vi "HumanExecute.vi"(8 "error in (no error)":errorcluster) -> (0 "error out":errorcluster)   [LabVIEW 2023]
doc: "Execute for Human\n\ninput:\n error in (cluster)\n\noutput:\n error out (cluster)"
uses:
  <vilib>/Rock Robotics/WPI/Joystick/XBox Buttons Indexer.ctl
  <vilib>/Rock Robotics/WPI/Joystick/XBox Axes Indexer.ctl
  <vilib>/Rock Robotics/WPI/ThirdParty/JAS_Junk/TrajLib/VI/BoolCmd_Send_Internal.vi
  <vilib>/Rock Robotics/WPI/ThirdParty/JAS_Junk/TrajLib/VI/BoolCmd_ObtainQueue.vi
  <vilib>/Rock Robotics/Network Tables/NT Write String.vi
  <vilib>/Rock Robotics/WPI/ThirdParty/JAS_Junk/TrajLib/Trajectory_Library.lvlib
  HumanGlobal.vi
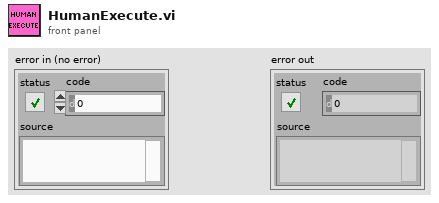
[diagram p1: front panel]
types:
  T1 = typedef "XBox Buttons Indexer.ctl" = enum16{"A", "B", "X", "Y", "Left Bumper", "Right Bumper", "Back", "Start", "Left Joystick", "Right Joystick"}
  T2 = typedef "XBox Axes Indexer.ctl" = enum16{"Left X", "Left Y", "Left Trigger", "Right Trigger", "Right X", "Right Y"}
  T3 = typedef "WPI_JoystickDevRef.ctl" = cluster{"Device":T4}
  T4 = typedef "WPI_JoystickDeviceEnum.ctl" = enum16{"USB 0", "USB 1", "USB 2", "USB 3", "USB 4", "USB 5"}
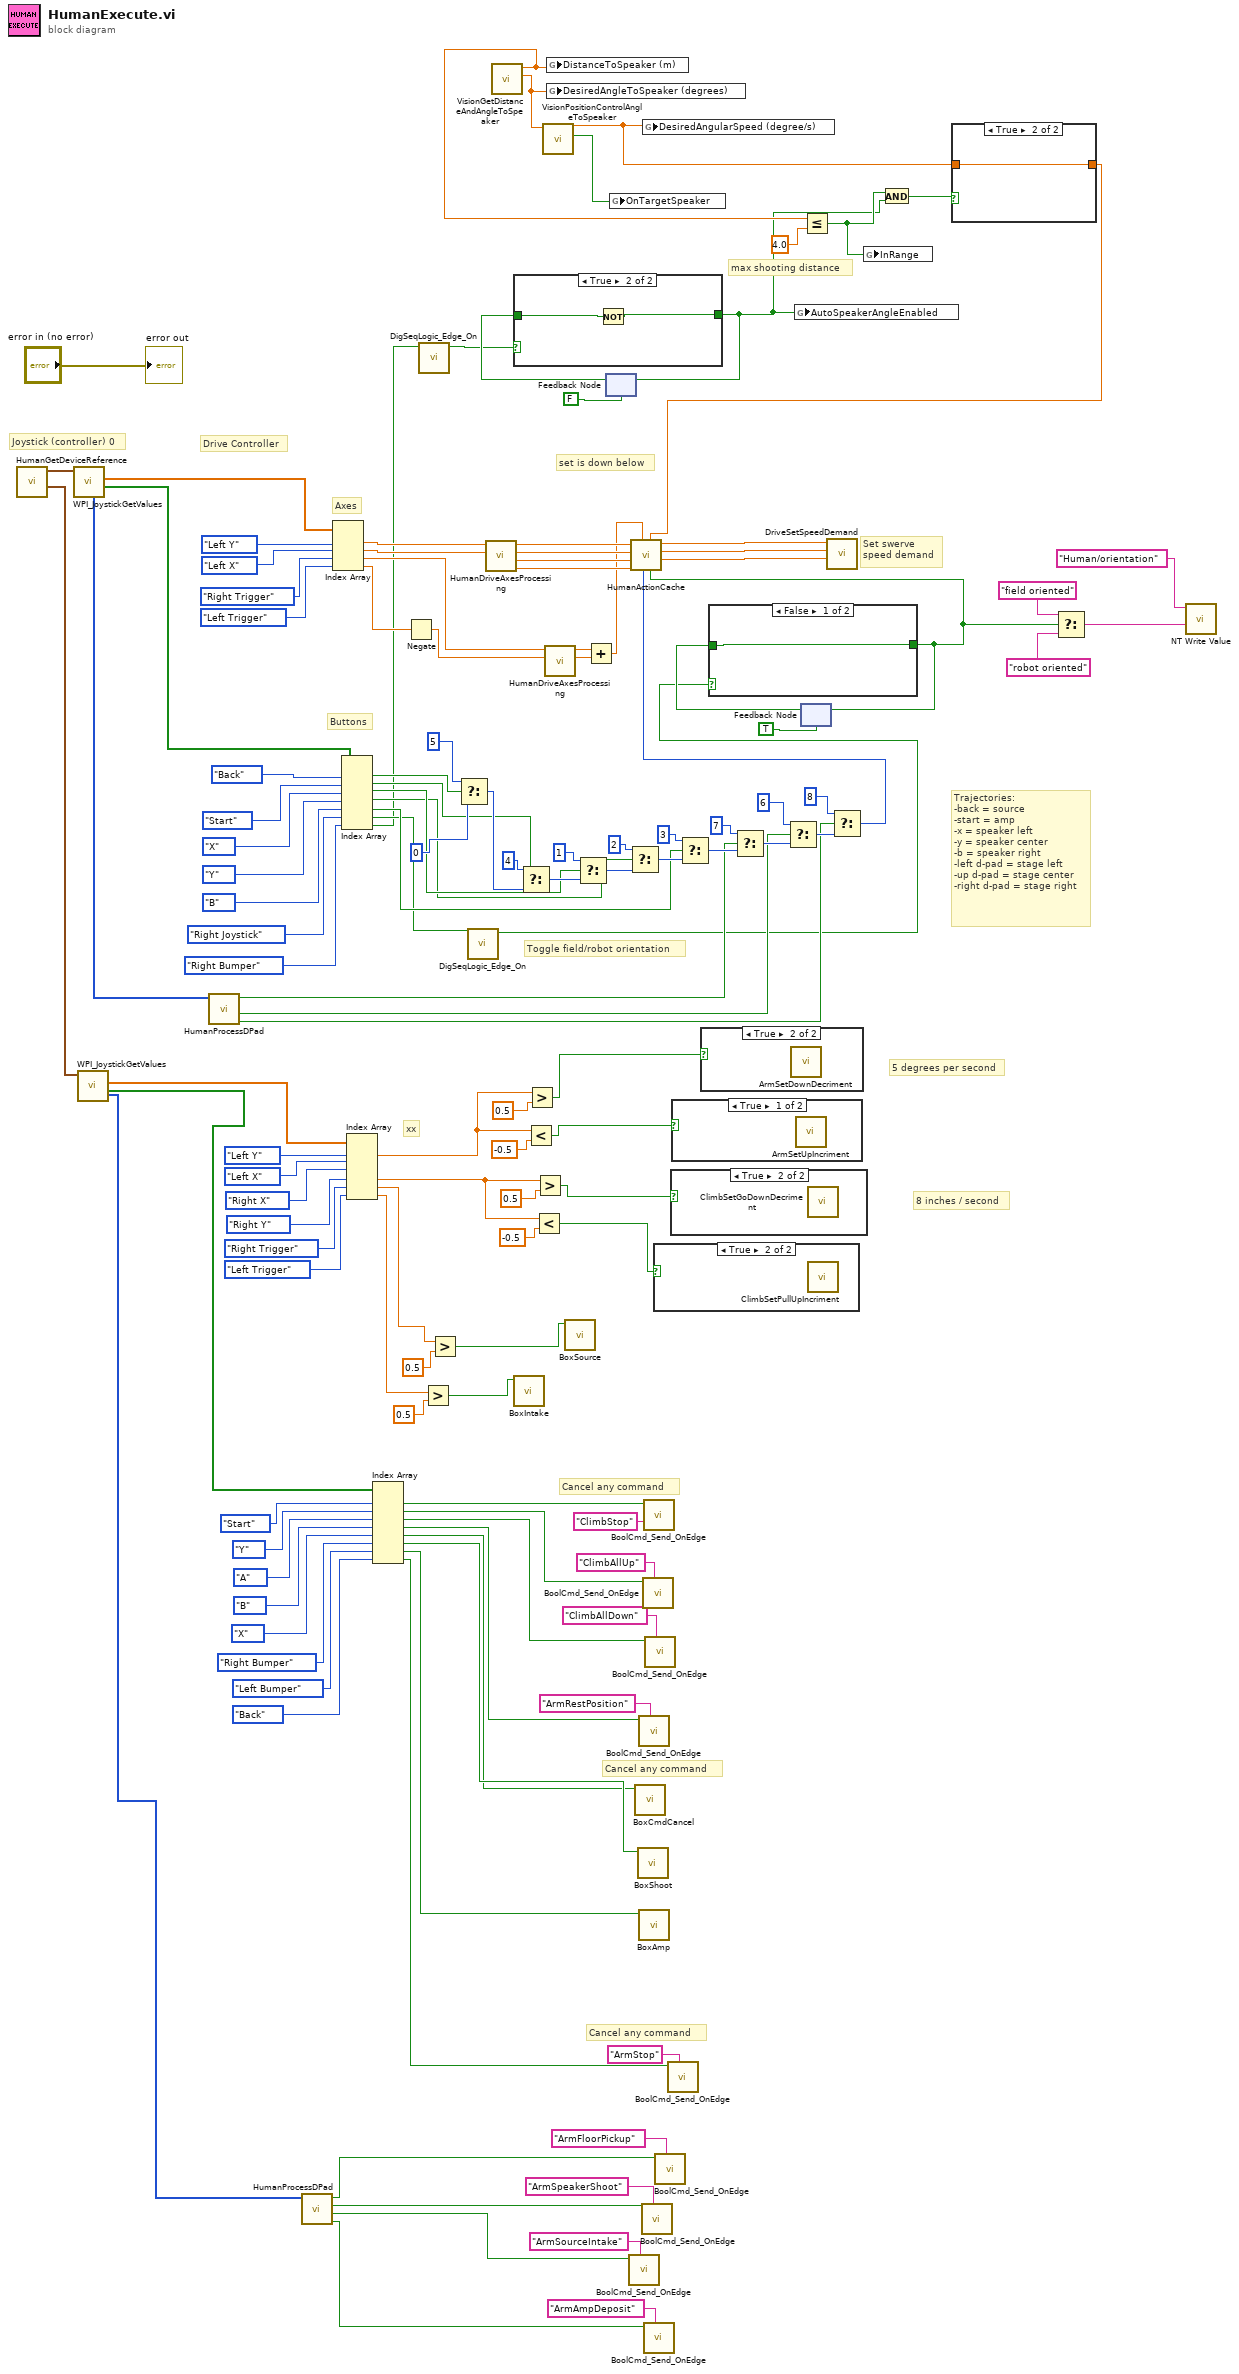
[diagram p0: block diagram]
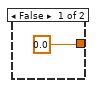
[diagram p3: hidden frame]
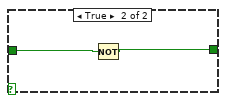
[diagram p4: hidden frame]
diagram:
  # "max shooting distance"
  # "Toggle field/robot orientation"
  # "8 inches / second"
  # "xx"
  # "Cancel any command"
  # "Cancel any command"
  # "5 degrees per second"
  # "Trajectories:\n-back = source\n-start = amp\n-x = speaker left\n-y = speaker center\n-b = speaker right\n-left d-pad = stage left\n-up d-pad = stage center\n-right d-pad = stage right"
  # "Buttons"
  # "Axes"
  # "Cancel any command"
  # "set is down below"
  # "Set swerve\nspeed demand"
  # "Joystick (controller) 0"
  # "Drive Controller"
  n1 = call "HumanGetDeviceReference.vi"() -> ("Aux Joy"=w112:T3, "Driver Joy"=w116:T3)  [unwired: 9 in, 1 out]
  n2 = call <vilib>:"WPI_JoystickGetValues.vi"("JoystickDevRef"=w116) -> ("Buttons"=w88:bool[], "Axes"=w98:dbl[], "POVs"=w130:i16[])  [unwired: 6 in, 2 out]
  n3 = call <vilib>:"WPI_JoystickGetValues.vi"("JoystickDevRef"=w112) -> ("Buttons"=w102:bool[], "Axes"=w111:dbl[], "POVs"=w59:i16[])  [unwired: 6 in, 2 out]
  n4 = call "HumanProcessDPad.vi"("POV"=w130) -> ("Right"=w37:bool, "Left"=w38:bool, "Up"=w39:bool)  [unwired: 7 in, 1 out]
  n5 = call "HumanProcessDPad.vi"("POV"=w59) -> ("Right"=w56:bool, "Left"=w54:bool, "Down"=w55:bool, "Up"=w57:bool)  [unwired: 7 in]
  n6 = Index Array(array=w98, index #1=XBox_Axes_Indexer."Left Y" ("XBox Axes"), index #2=XBox_Axes_Indexer."Left X" ("XBox Axes"), index #3=XBox_Axes_Indexer."Right Trigger" ("XBox Axes"), index #4=XBox_Axes_Indexer."Left Trigger" ("XBox Axes")) -> (element #1=w129:dbl, element #2=w128:dbl, element #3=w80:dbl, element #4=w79:dbl)
  n7 = Index Array(array=w88, index #1=XBox_Buttons_Indexer."Back" ("Nothing"), index #2=XBox_Buttons_Indexer."Start" ("Nothing"), index #3=XBox_Buttons_Indexer."X" ("Nothing"), index #4=XBox_Buttons_Indexer."Y" ("Nothing"), index #5=XBox_Buttons_Indexer."B" ("Nothing"), index #6=XBox_Buttons_Indexer."Right Joystick" ("Nothing"), index #7=XBox_Buttons_Indexer."Right Bumper" ("Nothing")) -> (element #1=w53:bool, element #2=w43:bool, element #3=w42:bool, element #4=w41:bool, element #5=w40:bool, element #6=w23:bool, element #7=w3:bool)
  n8 = Index Array(array=w111, index #1=XBox_Axes_Indexer."Left Y" ("XBox Axes"), index #2=XBox_Axes_Indexer."Left X" ("XBox Axes"), index #3=XBox_Axes_Indexer."Right X" ("XBox Axes"), index #4=XBox_Axes_Indexer."Right Y" ("XBox Axes"), index #5=XBox_Axes_Indexer."Right Trigger" ("XBox Axes"), index #6=XBox_Axes_Indexer."Left Trigger" ("XBox Axes")) -> (element #1=w73:dbl, element #4=w65:dbl, element #5=w96:dbl, element #6=w92:dbl)  [unwired: 2 out]
  n9 = Index Array "Index Array"(array=w102, index #1=XBox_Buttons_Indexer."Start" ("Nothing"), index #2=XBox_Buttons_Indexer."Y" ("OpenCloseClaw"), index #3=XBox_Buttons_Indexer."A" ("GrabberIn"), index #4=XBox_Buttons_Indexer."B" ("GrabberOut"), index #5=XBox_Buttons_Indexer."X" ("Nothing"), index #6=XBox_Buttons_Indexer."Right Bumper" ("Nothing"), index #7=XBox_Buttons_Indexer."Left Bumper" ("Nothing"), index #8=XBox_Buttons_Indexer."Back" ("Place Cone")) -> (element #1=w64:bool, element #2=w63:bool, element #3=w62:bool, element #4=w61:bool, element #5=w89:bool, element #6=w97:bool, element #7=w90:bool, element #8=w60:bool)
  n10 = Negate(x=w79) -> (-x=w125:dbl)
  n11 = call <vilib>:"DigSeqLogic_Edge_On.vi"("Input"=w3) -> ("On Edge"=w4:bool)  [unwired: 10 in]
  n12 = Greater?(x=w92, y=0.5) -> (0:w91:bool)
  n13 = Greater?(x=w96, y=0.5) -> (0:w94:bool)
  n14 = Select(t=5, s=w53, f=0) -> (s? t:f=w50:i32)
  n15 = call <vilib>:"DigSeqLogic_Edge_On.vi"("Input"=w23) -> ("On Edge"=w21:bool)  [unwired: 10 in]
  n16 = call "HumanDriveAxesProcessing.vi"("Left X"=w128, "Left Y"=w129) -> ("Right X"=w127:dbl, "Right Y"=w122:dbl, "Left X"=w126:dbl, "Left Y"=w121:dbl)  [unwired: 6 in]
  n17 = call "VisionGetDistanceAndAngleToSpeaker.vi"() -> ("DesiredAngle"=w14:dbl, "Distance"=w12:dbl)  [unwired: 10 in]
  n18 = call "BoxIntake.vi"("Box intake"=w91) -> ()  [unwired: 10 in, 1 out]
  n19 = Select(t=4, s=w43, f=w50) -> (s? t:f=w49:i32)
  n20 = Less?(x=w73, y=-0.5) -> (x < y?=w26:bool)
  n21 = Greater?(x=w73, y=0.5) -> (0:w25:bool)
  n22 = Less?(x=w65, y=-0.5) -> (x < y?=w28:bool)
  n23 = Greater?(x=w65, y=0.5) -> (0:w27:bool)
  n24 = call "VisionPositionControlAngleToSpeaker.vi"("TargetAngle"=w14) -> ("OnTargetSpeaker"=w13:bool, "DesiredAngularSpeed (degree/s)"=w10:dbl)  [unwired: 9 in]
  n25 = call "HumanDriveAxesProcessing.vi"("Left X"=w125, "Left Y"=w80) -> ("Left X"=w123:dbl, "Left Y"=w124:dbl)  [unwired: 6 in, 2 out]
  n26 = global write "HumanGlobal.vi" "DistanceToSpeaker (m)"(w12) -> ()
  n27 = global write "HumanGlobal.vi" "DesiredAngleToSpeaker (degrees)"(w14) -> ()
  n28 = call "BoxSource.vi"("Box source"=w94) -> ()  [unwired: 11 in]
  n29 = Select(t=1, s=w42, f=w49) -> (s? t:f=w48:i32)
  n30 = Add(x=w124, y=w123) -> (x+y=w120:dbl)
  n31 = feedback #1(FALSE) -> (w6:bool)
  n32 = case shown="True" w4 {
    tunnel: w6 -> [w134 w136]
    tunnel: [w134 w135] -> w2
    frame False {
    }
    frame True {
      n33 = Not(x=w136) -> (.not. x?=w135:bool)
    }
  }
  n34 = feedback-in #1(w2) -> ()
  n35 = global write "HumanGlobal.vi" "OnTargetSpeaker"(w13) -> ()
  n36 = call <vilib>:"BoolCmd_Send_OnEdge.vi"("Command Name"="ArmSourceIntake", "Value"=w54) -> ()  [unwired: 9 in, 1 out]
  n37 = Select(t=2, s=w41, f=w48) -> (s? t:f=w47:i32)
  n38 = call "BoxCmdCancel.vi"("box cancel"=w89) -> ()  [unwired: 11 in]
  n39 = call "BoxShoot.vi"("Box shoot"=w97) -> ()  [unwired: 10 in, 1 out]
  n40 = call <vilib>:"BoolCmd_Send_OnEdge.vi"("Command Name"="ArmRestPosition", "Value"=w61) -> ()  [unwired: 9 in, 1 out]
  n41 = call "BoxAmp.vi"("box amp"=w90) -> ()  [unwired: 11 in]
  n42 = call <vilib>:"BoolCmd_Send_OnEdge.vi"("Command Name"="ArmSpeakerShoot", "Value"=w55) -> ()  [unwired: 9 in, 1 out]
  n43 = global write "HumanGlobal.vi" "DesiredAngularSpeed (degree/s)"(w10) -> ()
  n44 = call <vilib>:"BoolCmd_Send_OnEdge.vi"("Command Name"="ClimbAllUp", "Value"=w63) -> ()  [unwired: 9 in, 1 out]
  n45 = call <vilib>:"BoolCmd_Send_OnEdge.vi"("Command Name"="ClimbStop", "Value"=w64) -> ()  [unwired: 9 in, 1 out]
  n46 = call <vilib>:"BoolCmd_Send_OnEdge.vi"("Command Name"="ArmAmpDeposit", "Value"=w56) -> ()  [unwired: 9 in, 1 out]
  n47 = call <vilib>:"BoolCmd_Send_OnEdge.vi"("Command Name"="ClimbAllDown", "Value"=w62) -> ()  [unwired: 9 in, 1 out]
  n48 = case shown="True" w28 {
    frame False {
    }
    frame True {
      n49 = call "ClimbSetPullUpIncriment.vi"() -> ()  [unwired: 11 in, 1 out]
    }
  }
  n50 = call <vilib>:"BoolCmd_Send_OnEdge.vi"("Command Name"="ArmFloorPickup", "Value"=w57) -> ()  [unwired: 9 in, 1 out]
  n51 = call <vilib>:"BoolCmd_Send_OnEdge.vi"("Command Name"="ArmStop", "Value"=w60) -> ()  [unwired: 9 in, 1 out]
  n52 = case shown="True" w27 {
    frame False {
    }
    frame True {
      n53 = call "ClimbSetGoDownDecriment.vi"() -> ()  [unwired: 11 in, 1 out]
    }
  }
  n54 = case shown="True" w26 {
    frame True {
      n55 = call "ArmSetUpIncriment.vi"() -> ()  [unwired: 11 in, 1 out]
    }
    frame False {
    }
  }
  n56 = Select(t=3, s=w40, f=w47) -> (s? t:f=w46:i32)
  n57 = case shown="True" w25 {
    frame False {
    }
    frame True {
      n58 = call "ArmSetDownDecriment.vi"() -> ()  [unwired: 11 in, 1 out]
    }
  }
  n59 = Select(t=7, s=w39, f=w46) -> (s? t:f=w45:i32)
  n60 = Select(t=6, s=w38, f=w45) -> (s? t:f=w44:i32)
  n61 = global write "HumanGlobal.vi" "AutoSpeakerAngleEnabled"(w2) -> ()
  n62 = feedback #2(TRUE) -> (w22:bool)
  n63 = case shown="False" w21 {
    tunnel: w22 -> [w137 w139]
    tunnel: [w137 w138] -> w19
    frame False {
    }
    frame True {
      n64 = Not(x=w139) -> (.not. x?=w138:bool)
    }
  }
  n65 = feedback-in #2(w19) -> ()
  n66 = Less Or Equal?(x=w12, y=4.0) -> (x <= y?=w9:bool)
  n67 = Select(t=8, s=w37, f=w44) -> (s? t:f=w29:i32)
  n68 = global write "HumanGlobal.vi" "InRange"(w9) -> ()
  n69 = And(x=w9, y=w2) -> (x .and. y?=w8:bool)
  n70 = case shown="True" w8 {
    tunnel: w10 -> [_ w141]
    tunnel: [0.0 w141] -> w1
    frame False {
    }
    frame True {
    }
  }
  n71 = call "HumanActionCache.vi"("Enable Field Oriented Drive"=w19, "AutoSpeakerAngle"=w1, "State"=w29, "Rotation"=w120, "Right X"=w127, "Right Y"=w122, "Left X"=w126, "Left Y"=w121) -> ("AMotorDemand"=w119:dbl, "YMotorDemand"=w118:dbl, "XMotorDemand"=w117:dbl)  [unwired: 1 in]
  n72 = call "DriveSetSpeedDemand.vi"("ASpeedDemand (d/s)"=w119, "YSpeedDemand (ft/s)"=w118, "XSpeedDemand (ft/s)"=w117) -> ()  [unwired: 9 in]
  n73 = Select(t="field oriented", s=w19, f="robot oriented") -> (s? t:f=w16:string)
  n74 = call-poly <vilib>:"NT Write Value.vi"("value"=w16, "name"="Human/orientation") -> ()  [unwired: 9 in, 1 out]
  "error out" <- "error in (no error)"
